vi "pressure_ut_test_gauge_small_window.vi"(8 "Error In":errorcluster, 11 "Manometr in":T2) -> (0 "Error Out":errorcluster, 3 "Manometr out":T2)   [LabVIEW 2018]
uses:
  PressureGaugeInfo.ctl
  <vilib>/Utility/miscctls.llb/LVDateTimeRec.ctl
  MOKO_LabViewLibrary/MokoSTM/MokoClassicUtilitySTM/MCUS_STM.ctl
  MOKO_LabViewLibrary/MokoSTM/MokoClassicUtilitySTM/MCUS_ITEM.ctl
panel:
  in  "Минимальное значение":i64 caption="Минимальное значение на шкале прибора:"
  in  "Наименование СИ:":string
  in  "Производственный № прибора:":string
  in  "Пределы допускаемой погрешости D=±:":dbl min=0.0 format="%#_4f"
  in  "№ прибора:":dbl
  out "date time rec":T1
  in  "Драйвер:":string(combo)="0,4"
  in  "№ протокола":string caption="№ протокола:"
  in  "ММ":string(combo)
  in  "ДД":i64=1 min=1 max=31
  in  "ГГГГ":dbl=1.0 caption="ГГГГ:"
  in  "Давление":dbl caption="Давление окружающей среды, мм. рт. ст.:"
  in  "Цена деления":dbl caption="Цена деления:" format="%#_4g"
  in  "Температура":dbl caption="Температура окружающего воздуха, °С:"
  in  "Влажность":dbl caption="Относительная влажность воздуха, %:"
  in  "Номер заказа":string caption="Номер заказа:"
  in  "Номер рабочего места":string caption="Номер рабочего места:"
  in  "ФИО":string caption="Поверку провел:"
  in  "Место проведения":string caption="Место проведения поверки:"
  in  "Владелец":string caption="Владелец:"
  in  "Номер клейма":string caption="Номер клейма:"
  in  "Тип":string caption="Тип:"
  in  "Первая точка":dbl=1.0 caption="Первая поверяемая точка на шкале прибора после нуля:" format="%#_3f"
  in  "Предельное давление":dbl=1.0 caption="Предельное значение давления на шкале прибора:" format="%#_3f"
  in  "Класс точности:":string(combo)="0,4"
  in  "Единица измерения:":string(combo)="kPa"
  in  "Применить":bool
  # "!\"№;%:?*()_+ЙЦУКЕНГ?*Ш(ЩЗХЪ\nФЫВАПРОЛДЖЭ\nЯЧСМИТЬБЮ,"
  # "Информация об образце"
  # "Информация о поверке"
  # "0,4\n0,6\n1\n1,5\n1,6\n2,5\n4"
  # "kPa\nbar\nkgf/cm2\nMPa"
  # "Характеристики манометра"
  # "Условия поверки"
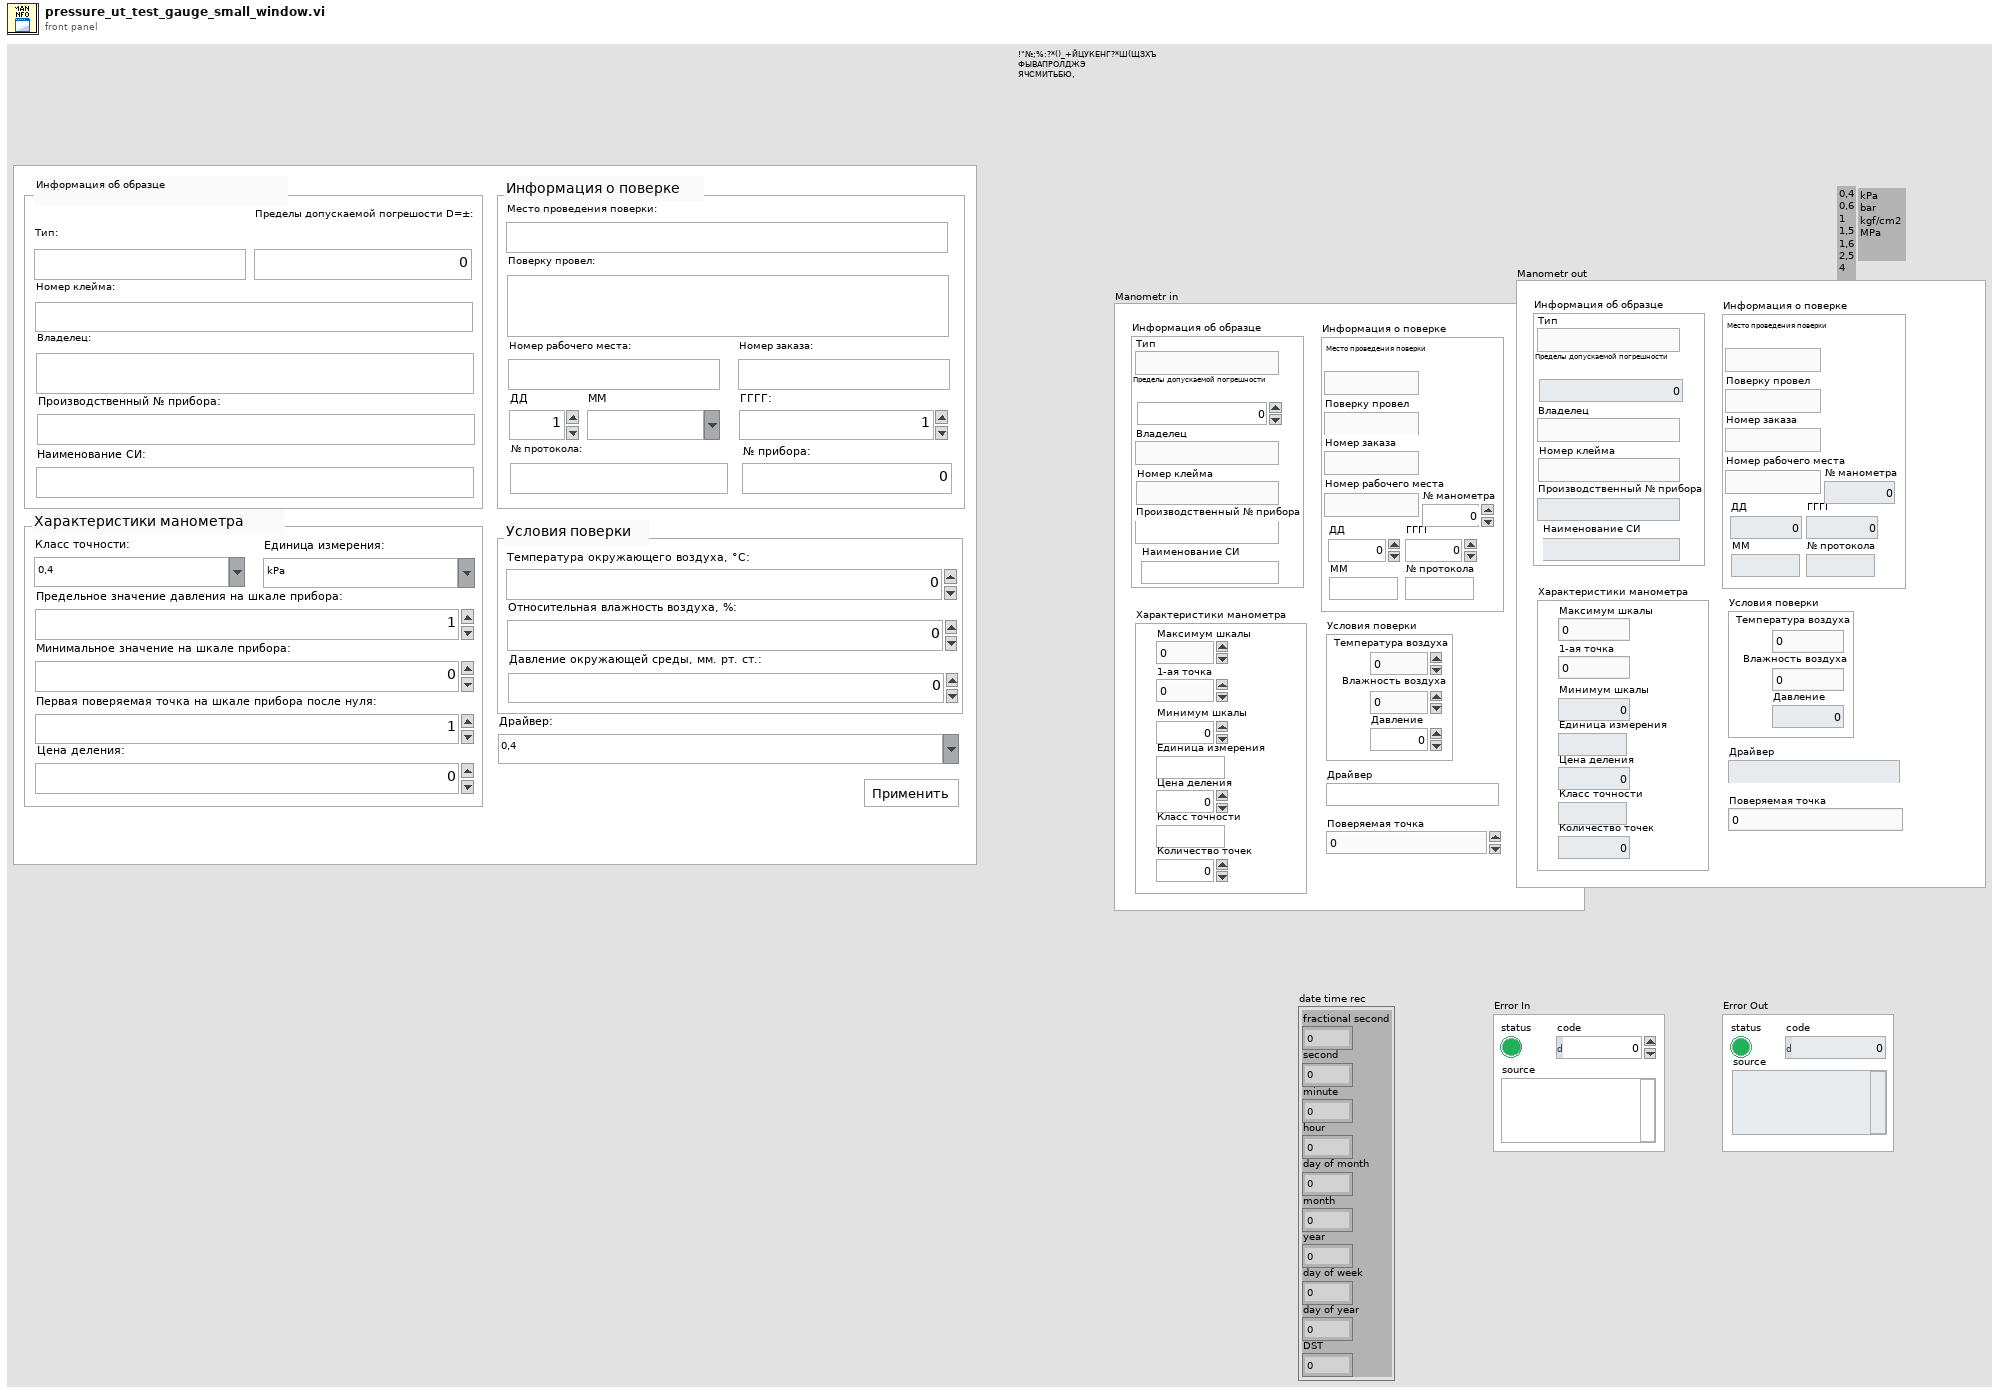
[diagram p1: front panel]
types:
  T1 = typedef "LVDateTimeRec.ctl" = cluster{"fractional second":dbl, "second":i32, "minute":i32, "hour":i32, "day of month":i32, "month":i32, "year":i32, "day of week":i32, "day of year":i32, "DST":i32}
  T2 = typedef "PressureGaugeInfo.ctl" = cluster{"Информация об образце":cluster{"Тип":string, "Владелец":string, "Номер клейма":string, "Пределы допускаемой погрешности ":dbl, "Производственный № прибора":string, "Наименование СИ":string}, "Информация о поверке":cluster{"Место проведения поверки":string, "Поверку провел":string, "Номер заказа":string, "Номер рабочего места":string, "ДД":dbl, "ММ":string, "ГГГГ":dbl, "№ протокола":string, "№ манометра":dbl}, "Характеристики манометра":cluster{"Максимум шкалы":dbl, "1-ая точка":dbl, "Единица измерения":string, "Цена деления":dbl, "Класс точности":string, "Минимум шкалы":dbl, "Количество точек":dbl}, "Условия поверки":cluster{"Температура воздуха":dbl, "Влажность воздуха":dbl, "Давление":dbl}, "Драйвер":string, "Поверяемая точка":dbl}
  T3 = typedef "MCUS_STM.ctl" = cluster{"main stm":T4, "data":string}
  T4 = typedef "MCUS_ITEM.ctl" = enum16{"idle", "_____ main_____ ", "Init", "Stop", "Apply values"}
  T5 = cluster{"Максимум шкалы":dbl, "1-ая точка":dbl, "Единица измерения":string, "Цена деления":dbl, "Класс точности":string, "Минимум шкалы":dbl, "Количество точек":dbl}
  T6 = cluster{"Температура воздуха":dbl, "Влажность воздуха":dbl, "Давление":dbl}
  T7 = cluster{"Тип":string, "Владелец":string, "Номер клейма":string, "Пределы допускаемой погрешности ":dbl, "Производственный № прибора":string, "Наименование СИ":string}
  T8 = cluster{"Место проведения поверки":string, "Поверку провел":string, "Номер заказа":string, "Номер рабочего места":string, "ДД":dbl, "ММ":string, "ГГГГ":dbl, "№ протокола":string, "№ манометра":dbl}
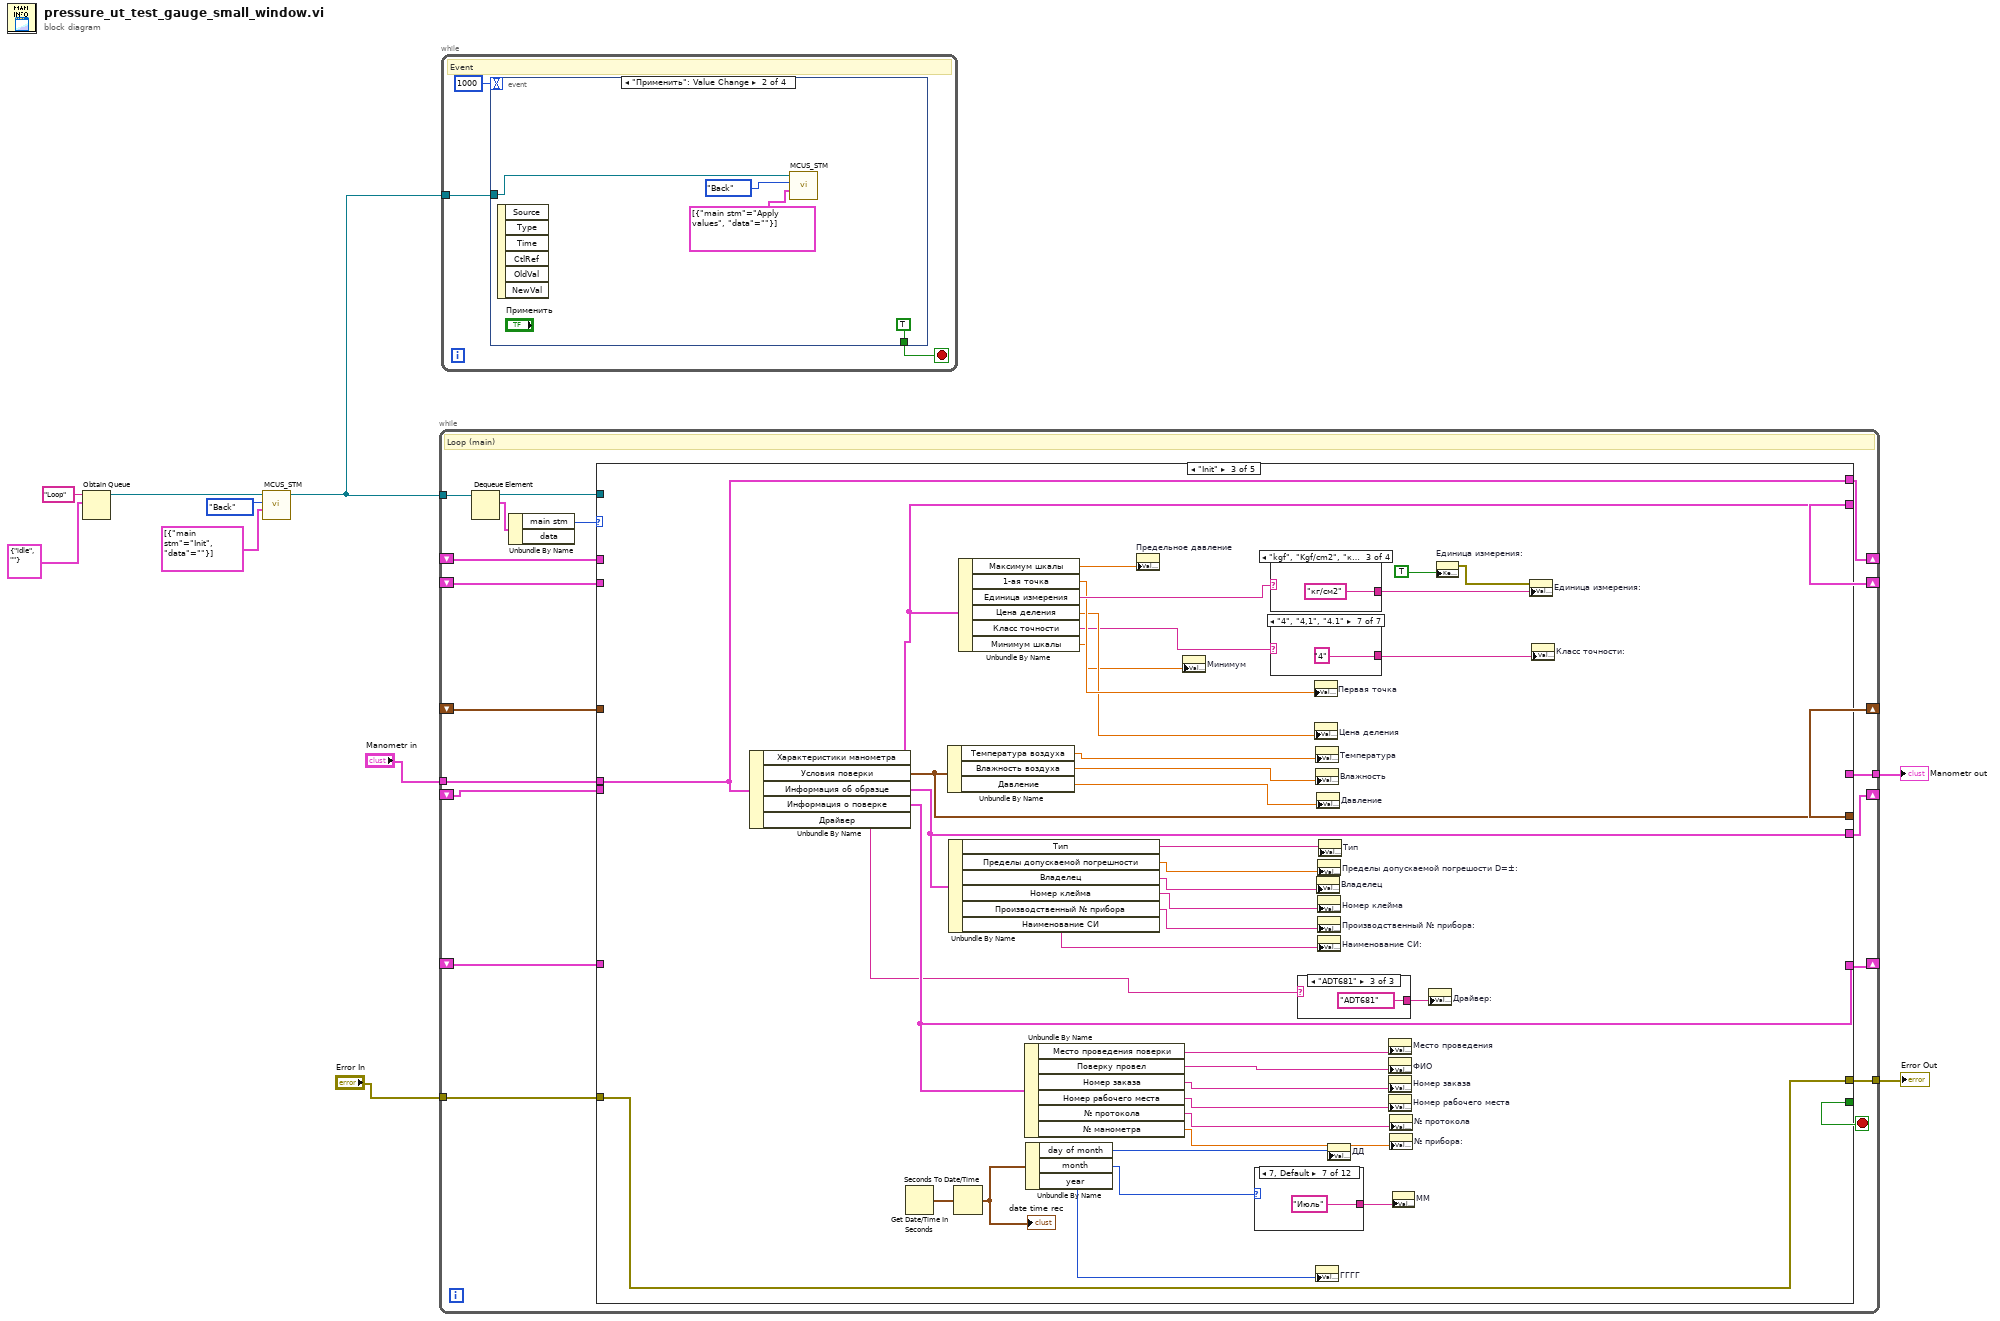
[diagram p0: block diagram]
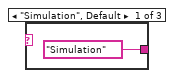
[diagram p4: hidden frame]
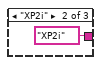
[diagram p5: hidden frame]
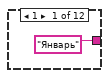
[diagram p6: hidden frame]
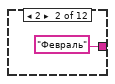
[diagram p7: hidden frame]
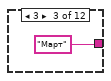
[diagram p8: hidden frame]
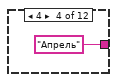
[diagram p9: hidden frame]
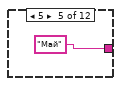
[diagram p10: hidden frame]
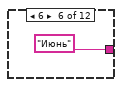
[diagram p11: hidden frame]
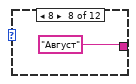
[diagram p12: hidden frame]
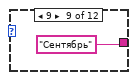
[diagram p13: hidden frame]
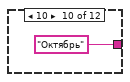
[diagram p14: hidden frame]
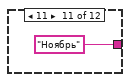
[diagram p15: hidden frame]
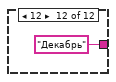
[diagram p16: hidden frame]
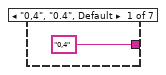
[diagram p17: hidden frame]
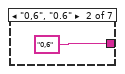
[diagram p18: hidden frame]
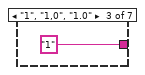
[diagram p19: hidden frame]
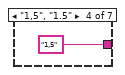
[diagram p20: hidden frame]
diagram:
  n1 = Obtain Queue(name (unnamed)="Loop", element data type=T3 {"main stm"=enum."idle", "data"=""} ("MOKO_NMEA")) -> (queue out=w10:refnum<queue>)  [unwired: 3 in, 2 out]
  n2 = call "MCUS_STM.vi"("StateMachineSteps"=T3[] [{"main stm"=enum."Init", "data"=""}], "FNs"=enum16{"Back", "Front", "Replace"}."Back", "Queue in"=w10) -> ("Queue out"=w5:refnum<queue>)  [unwired: 7 in, 1 out]
  n3 = while {
    tunnel: w5 -> [w29]
    shift-right: [w25] -> _
    shift-left: _ -> [w24]
    shift-right: [w23] -> _
    shift-left: _ -> [w22]
    shift-right: [w21] -> _
    shift-left: _ -> [w20]
    shift-right: [w19] -> _
    shift-left: _ -> [w18]
    shift-right: [w17] -> _
    shift-left: _ -> [w15]
    tunnel: [w14] -> w4
    tunnel: "Manometr in" -> [w13]
    tunnel: "Error In" -> [w12]
    tunnel: [w11] -> w1
    stop <- w16 stop-if-true
    # "Loop (main)"
    n4 = Dequeue Element(queue=w29) -> (queue out=w28:refnum<queue>, element=w27:T3)  [unwired: 2 in, 2 out]
    n5 = Unbundle By Name(w27) -> ("main stm"=w26:T4)  [unwired: 1 out]
    n6 = case shown="\"Init\"" w26 {
      tunnel: w28 -> [_ _ _ _ _]
      tunnel: [w33 _ w45 _ w142] -> w25
      tunnel: w24 -> [w33 _ _ w109 w142]
      tunnel: [w32 _ w59 _ w141] -> w23
      tunnel: w22 -> [w32 _ _ w124 w141]
      tunnel: [w31 _ w58 _ w139] -> w21
      tunnel: w20 -> [w31 _ _ w123 w139]
      tunnel: [w30 _ w57 _ w138] -> w19
      tunnel: w18 -> [w30 _ _ w122 w138]
      tunnel: [w34 _ w56 _ w143] -> w17
      tunnel: w15 -> [w34 _ _ w120 w143]
      tunnel: [_ _ _ TRUE TRUE] -> w16
      tunnel: [_ _ _ w118 w140] -> w14
      tunnel: w13 -> [_ _ w56 _ w140]
      tunnel: w12 -> [_ _ w55 w117 w137]
      tunnel: [_ _ w55 w117 w137] -> w11
      frame "idle", Default {
      }
      frame "_____ main_____ " {
      }
      frame "Init" {
        n7 = Unbundle By Name(w56) -> ("Характеристики манометра"=w45:T5, "Условия поверки"=w59:T6, "Информация об образце"=w58:T7, "Информация о поверке"=w57:T8, "Драйвер"=w38:string)
        n8 = Get Date/Time In Seconds() -> (seconds since 1Jan1904=w53:timestamp)
        n9 = Unbundle By Name(w59) -> ("Температура воздуха"=w70:dbl, "Влажность воздуха"=w69:dbl, "Давление"=w68:dbl)
        n10 = Unbundle By Name(w58) -> ("Тип"=w66:string, "Пределы допускаемой погрешности"=w46:dbl, "Владелец"=w65:string, "Номер клейма"=w64:string, "Производственный № прибора"=w36:string, "Наименование СИ"=w35:string)
        n11 = Seconds To Date/Time(time stamp (now)=w53) -> (date time rec=w52:T1)  [unwired: 1 in]
        "date time rec" <- w52
        n12 = Unbundle By Name(w45) -> ("Максимум шкалы"=w44:dbl, "1-ая точка"=w42:dbl, "Единица измерения"=w43:string, "Цена деления"=w41:dbl, "Класс точности"=w40:string, "Минимум шкалы"=w39:dbl)
        n13 = Unbundle By Name(w57) -> ("Место проведения поверки"=w63:string, "Поверку провел"=w62:string, "Номер заказа"=w61:string, "Номер рабочего места"=w60:string, "№ протокола"=w54:string, "№ манометра"=w47:dbl)
        n14 = Unbundle By Name(w52) -> ("day of month"=w51:i32, "month"=w50:i32, "year"=w48:i32)
        n15 = property on="Предельное давление" class="DigNum (strict)"("Value"=w44) -> ()  [unwired: 2 in, 2 out]
        n16 = property on="Минимум" class="DigNum (strict)"("Val(Sgnl)"=w39) -> ()  [unwired: 2 in, 2 out]
        n17 = case shown="7, Default" w50 {
          tunnel: ["Январь" "Февраль" "Март" "Апрель" "Май" "Июнь" "Июль" "Август" "Сентябрь" "Октябрь" "Ноябрь" "Декабрь"] -> w49
          frame 1 {
          }
          frame 2 {
          }
          frame 3 {
          }
          frame 4 {
          }
          frame 5 {
          }
          frame 6 {
          }
          frame 7, Default {
          }
          frame 8 {
          }
          frame 9 {
          }
          frame 10 {
          }
          frame 11 {
          }
          frame 12 {
          }
        }
        n18 = case shown="\"kgf\", \"Kgf/cm2\", \"кг/см2\"" w43 {
          tunnel: ["кПа" "бар" "кг/см2" "МПа"] -> w73
          frame "kpa", "кпа", Default {
          }
          frame "bar", "бар" {
          }
          frame "kgf", "Kgf/cm2", "кг/см2" {
          }
          frame "mpa", "мпа" {
          }
        }
        n19 = case shown="\"4\", \"4,1\", \"4.1\"" w40 {
          tunnel: ["0,4" "0,6" "1" "1,5" "1,6" "2,5" "4"] -> w67
          frame "0,4", "0.4", Default {
          }
          frame "0,6", "0.6" {
          }
          frame "1", "1,0", "1.0" {
          }
          frame "1,5", "1.5" {
          }
          frame "1,6", "1.6" {
          }
          frame "2,5", "2.5" {
          }
          frame "4", "4,1", "4.1" {
          }
        }
        n20 = case shown="\"ADT681\"" w38 {
          tunnel: ["Simulation" ("Драйвер:") "XP2i" ("Драйвер:") "ADT681" ("Драйвер:")] -> w37
          frame "Simulation", Default {
          }
          frame "XP2i" {
          }
          frame "ADT681" {
          }
        }
        n21 = property on="Первая точка" class="DigNum (strict)"("Value"=w42) -> ()  [unwired: 2 in, 2 out]
        n22 = property on="Цена деления" class="DigNum (strict)"("Value"=w41) -> ()  [unwired: 2 in, 2 out]
        n23 = property on="Температура" class="DigNum (strict)"("Value"=w70) -> ()  [unwired: 2 in, 2 out]
        n24 = property on="Влажность" class="DigNum (strict)"("Value"=w69) -> ()  [unwired: 2 in, 2 out]
        n25 = property on="ГГГГ" class="DigNum (strict)"("Value"=w48) -> ()  [unwired: 2 in, 2 out]
        n26 = property on="Давление" class="DigNum (strict)"("Value"=w68) -> ()  [unwired: 2 in, 2 out]
        n27 = property on="Владелец" class="Str"("Value"=w65) -> ()  [unwired: 2 in, 2 out]
        n28 = property on="Пределы допускаемой погрешости D=±:" class="DigNum (strict)"("Val(Sgnl)"=w46) -> ()  [unwired: 2 in, 2 out]
        n29 = property on="Номер клейма" class="Str"("Value"=w64) -> ()  [unwired: 2 in, 2 out]
        n30 = property on="Производственный № прибора:" class="Str"("Value"=w36) -> ()  [unwired: 2 in, 2 out]
        n31 = property on="Наименование СИ:" class="Str"("Value"=w35) -> ()  [unwired: 2 in, 2 out]
        n32 = property on="Тип" class="Str"("Value"=w66) -> ()  [unwired: 2 in, 2 out]
        n33 = property on="ДД" class="DigNum (strict)"("Value"=w51) -> ()  [unwired: 2 in, 2 out]
        n34 = property on="Место проведения" class="Str"("Value"=w63) -> ()  [unwired: 2 in, 2 out]
        n35 = property on="ФИО" class="Str"("Value"=w62) -> ()  [unwired: 2 in, 2 out]
        n36 = property on="Номер заказа" class="Str"("Value"=w61) -> ()  [unwired: 2 in, 2 out]
        n37 = property on="Номер рабочего места" class="Str"("Value"=w60) -> ()  [unwired: 2 in, 2 out]
        n38 = property on="№ протокола" class="Str"("Value"=w54) -> ()  [unwired: 2 in, 2 out]
        n39 = property on="№ прибора:" class="DigNum (strict)"("Value"=w47) -> ()  [unwired: 2 in, 2 out]
        n40 = property on="ММ" class="CmbBox"("Value"=w49) -> ()  [unwired: 2 in, 2 out]
        n41 = property on="Драйвер:" class="CmbBox"("Value"=w37) -> ()  [unwired: 2 in, 2 out]
        n42 = property on="Единица измерения:" class="CmbBox"("Key Focus"=TRUE) -> (error out=w71:errorcluster)  [unwired: 2 in, 1 out]
        n43 = property on="Единица измерения:" class="CmbBox"(error in=w71, "Value"=w73) -> ()  [unwired: 1 in, 2 out]
        n44 = property on="Класс точности:" class="CmbBox"("Value"=w67) -> ()  [unwired: 2 in, 2 out]
      }
      frame "Apply values" {
        n45 = Bundle By Name(cluster=w123, "Тип"="Тип", "Пределы допускаемой погрешности"="Пределы допускаемой погрешости D=±:", "Владелец"="Владелец", "Номер клейма"="Номер клейма", "Производственный № прибора"="Производственный № прибора:", "Наименование СИ"="Наименование СИ:") -> (w132:T7)
        n46 = Bundle By Name(cluster=w122, "Место проведения поверки"="Место проведения", "Поверку провел"="ФИО", "Номер заказа"="Номер заказа", "Номер рабочего места"="Номер рабочего места", "ДД"="ДД", "ММ"="ММ", "ГГГГ"="ГГГГ", "№ протокола"="№ протокола", "№ манометра"="№ прибора:") -> (w121:T8)
        n47 = Bundle By Name(cluster=w124, "Температура воздуха"="Температура", "Влажность воздуха"="Влажность", "Давление"="Давление") -> (w133:T6)
        n48 = Bundle By Name(cluster=w109, "Максимум шкалы"="Предельное давление", "1-ая точка"="Первая точка", "Единица измерения"="Единица измерения:", "Цена деления"="Цена деления", "Класс точности"="Класс точности:", "Минимум шкалы"="Минимальное значение") -> (w108:T5)
        n49 = Bundle By Name(cluster=w120, "Характеристики манометра"=w108, "Условия поверки"=w133, "Информация об образце"=w132, "Информация о поверке"=w121, "Драйвер"="Драйвер:") -> (w118:T2)
      }
      frame "Stop" {
      }
    }
  }
  "Manometr out" <- w4
  "Error Out" <- w1
  n50 = while {
    tunnel: w5 -> [w145]
    stop <- w147 stop-if-true
    # "Event"
    n51 = event shown="[1] \"Применить\": Value Change" {
      selector: _ -> [_ _ _ _]
      dyn-events: _ -> [_ _ _ _]
      timeout: 1000 -> [_ _ _ _]
      tunnel: [_ TRUE _ TRUE] -> w147
      tunnel: w145 -> [_ w150 _ w152]
      event Timeout {
        n52 = event-data() -> ()  [unwired: 1 in, 3 out]
      }
      event "Применить": Value Change {
        n53 = event-data() -> ()  [unwired: 1 in, 6 out]
        n54 = call "MCUS_STM.vi"("StateMachineSteps"=T3[] [{"main stm"=enum."Apply values", "data"=""}], "FNs"=enum16{"Back", "Front", "Replace"}."Back", "Queue in"=w150) -> ()  [unwired: 7 in, 2 out]
      }
      event "Единица измерения:", "Класс точности:", "Предельное давление", "Первая точка", "Тип", "Номер клейма", "Владелец", "Место проведения", "ФИО", "Номер рабочего места", "Номер заказа", "Влажность", "Температура", "Цена деления", "Давление", "ГГГГ", "ДД", "ММ": Value Change {
        n55 = event-data() -> ()  [unwired: 1 in, 6 out]
      }
      event Panel Close {
        n56 = event-data() -> ()  [unwired: 1 in, 4 out]
        n57 = call "MCUS_STM.vi"("StateMachineSteps"=T3[] [{"main stm"=enum."Stop", "data"=""}], "FNs"=enum16{"Back", "Front", "Replace"}."Replace", "Queue in"=w152) -> ()  [unwired: 7 in, 2 out]
      }
    }
  }
